vi "CLD 4 Event Structure Time Out Front Panel.vi"() -> ()   [LabVIEW 2018]
doc: "CLD 4 exercise"
uses:
  States.ctl
panel:
  in  "Decrement":bool
  out "Error Out":errorcluster
  in  "Error In":errorcluster
  out "Time Has Elapsed":bool
  out "Count":string="0"
  in  "Increment":bool
  in  "Stop VI":bool
  in  "Timeout Target (s)":dbl=2.0
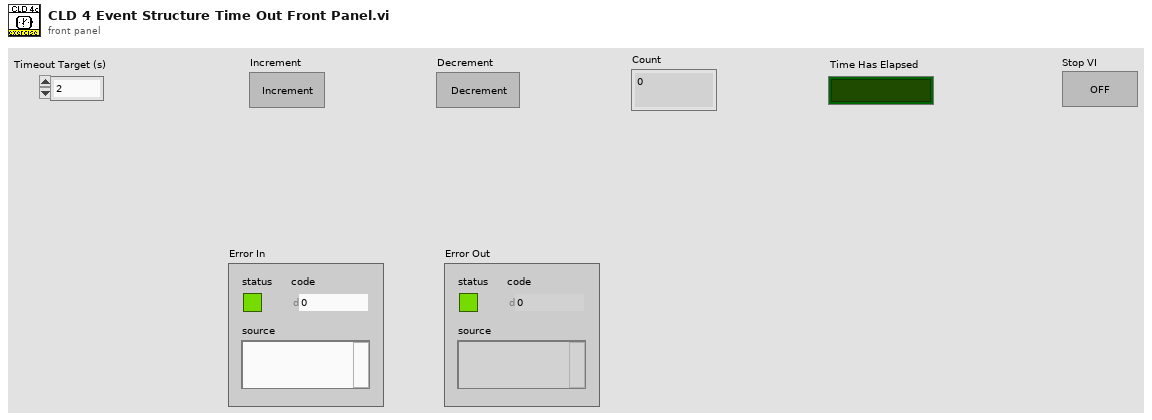
[diagram p1: front panel]
types:
  T1 = typedef "States.ctl" = enum16{"Update Target", "Wait for Event", "Inicialize", "Increment", "Decrement", "Time Has Elapsed", "Stop"}
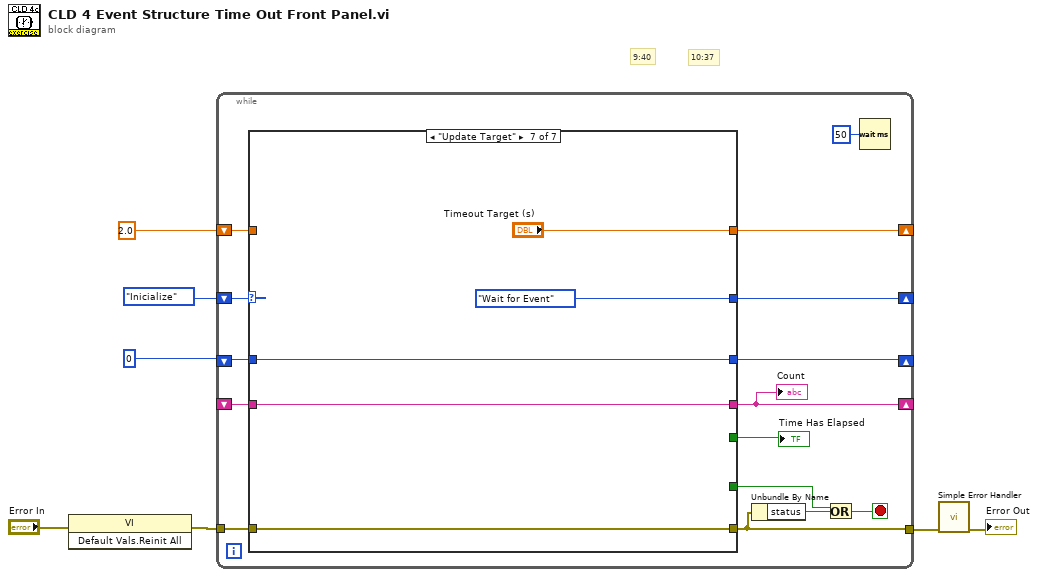
[diagram p0: block diagram]
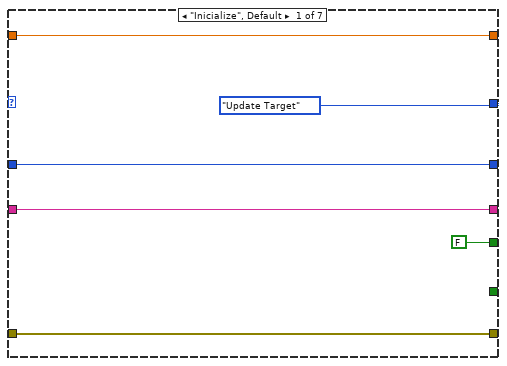
[diagram p2: hidden frame]
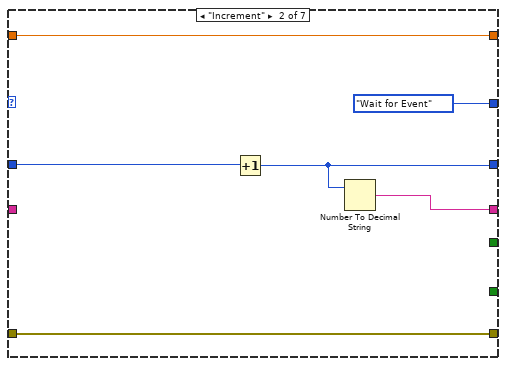
[diagram p3: hidden frame]
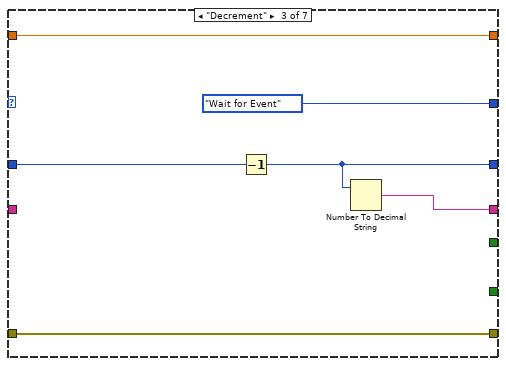
[diagram p4: hidden frame]
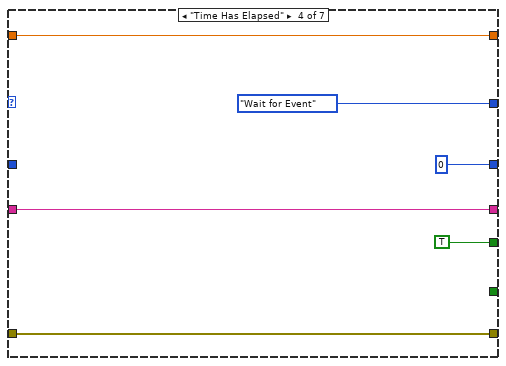
[diagram p5: hidden frame]
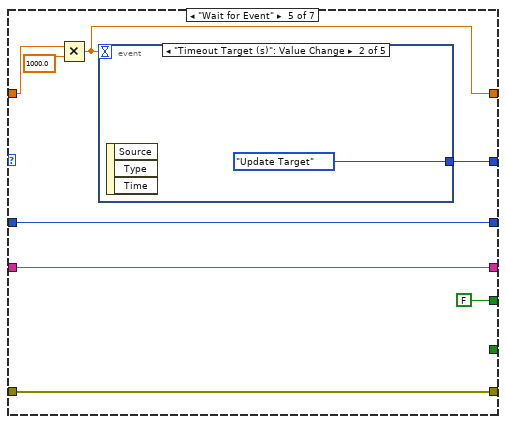
[diagram p6: hidden frame]
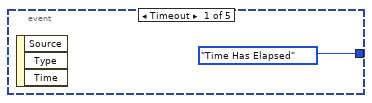
[diagram p7: hidden frame]
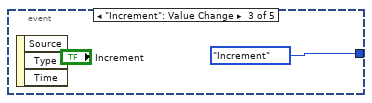
[diagram p8: hidden frame]
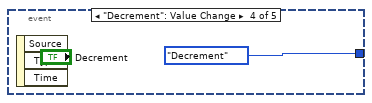
[diagram p9: hidden frame]
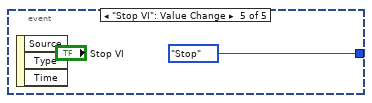
[diagram p10: hidden frame]
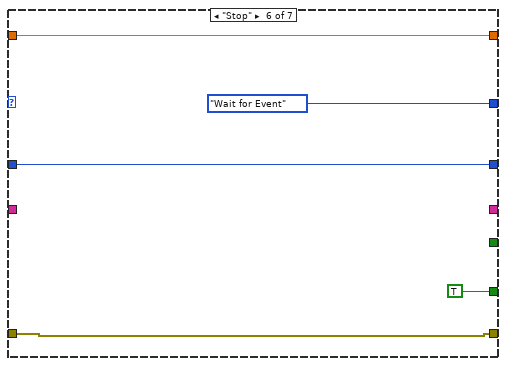
[diagram p11: hidden frame]
diagram:
  # "9:40"
  # "10:37"
  n1 = invoke class="VI" method="Default Vals.Reinit All"(error in="Error In") -> (error out=w2:errorcluster)  [unwired: 2 in, 2 out]
  n2 = while {
    shift-right: [w21] -> _
    shift-left: States."Inicialize" -> [w22]
    shift-right: [w18] -> _
    shift-left: u32 0 -> [w19]
    shift-right: [w17] -> _
    shift-left: _ -> [w16]
    tunnel: w2 -> [w15]
    tunnel: [w11] -> w5
    shift-right: [w9] -> _
    shift-left: 2.0 ("Timeout Target (s)") -> [w8]
    stop <- w14 stop-if-true
    n3 = case shown="\"Update Target\"" w22 {
      tunnel: [States."Update Target" States."Wait for Event" States."Wait for Event" States."Wait for Event" w54 States."Wait for Event" States."Wait for Event"] -> w21
      tunnel: [FALSE _ _ TRUE FALSE _ _] -> w20
      tunnel: [w26 w32 w38 w44 w52 _ w66] -> w17
      tunnel: w19 -> [w25 w34 w40 _ w53 w62 w67]
      tunnel: [w25 w33 w39 u32 0 w53 w62 w67] -> w18
      tunnel: [_ _ _ _ _ TRUE _] -> w13
      tunnel: w16 -> [w26 _ _ w44 w52 _ w66]
      tunnel: w15 -> [w24 w30 w36 w42 w51 w61 w69]
      tunnel: [w24 w30 w36 w42 w51 w61 w69] -> w11
      tunnel: [w23 w29 w35 w41 w47 w60 "Timeout Target (s)"] -> w9
      tunnel: w8 -> [w23 w29 w35 w41 w49 w60 _]
      frame "Inicialize", Default {
      }
      frame "Increment" {
        n4 = Increment(x=w34) -> (x+1=w33:u32)
        n5 = Number To Decimal String(number=w33) -> (decimal integer string=w32:string)  [unwired: 1 in]
      }
      frame "Decrement" {
        n6 = Decrement(x=w40) -> (x-1=w39:u32)
        n7 = Number To Decimal String(number=w39) -> (decimal integer string=w38:string)  [unwired: 1 in]
      }
      frame "Time Has Elapsed" {
      }
      frame "Wait for Event" {
        n8 = Multiply(x=w49, y=1000.0) -> (x*y=w47:dbl)
        n9 = event shown="[1] \"Timeout Target (s)\": Value Change" {
          selector: _ -> [_ _ _ _ _]
          dyn-events: _ -> [_ _ _ _ _]
          timeout: w47 -> [_ _ _ _ _]
          tunnel: [States."Time Has Elapsed" States."Update Target" States."Increment" States."Decrement" States."Stop"] -> w54
          event Timeout {
            n10 = event-data() -> ()  [unwired: 1 in, 3 out]
          }
          event "Timeout Target (s)": Value Change {
            n11 = event-data() -> ()  [unwired: 1 in, 3 out]
          }
          event "Increment": Value Change {
            n12 = event-data() -> ()  [unwired: 1 in, 3 out]
          }
          event "Decrement": Value Change {
            n13 = event-data() -> ()  [unwired: 1 in, 3 out]
          }
          event "Stop VI": Value Change {
            n14 = event-data() -> ()  [unwired: 1 in, 3 out]
          }
        }
      }
      frame "Stop" {
      }
      frame "Update Target" {
      }
    }
    "Time Has Elapsed" <- w20
    "Count" <- w17
    n15 = Unbundle By Name(w11) -> ("status"=w12:bool)
    n16 = Or(x=w13, y=w12) -> (x .or. y?=w14:bool)
    n17 = Wait (ms)(milliseconds to wait=u32 50) -> ()  [unwired: 1 out]
  }
  n18 = call <vilib>:"Simple Error Handler.vi"("error in (no error)"=w5) -> ("error out"=→"Error Out":errorcluster)  [unwired: 4 in, 4 out]
